vi "Auto Check Each Tube Posibly Modded for Prevent Trip.vi"(6 "error in (no error)":errorcluster, 8 "BoardHandle in":T1, 9 "Barcodes in":string[](array[string]), 10 "Tube #":i32) -> (0 "BoardHandle out":T1, 1 "error out":errorcluster, 2 "channel 4 currents":dbl[](array[numeric]), 3 "Actual Voltage Level (V) 2":dbl format="%#_13g", 5 "channel 3 currents":dbl[](array[numeric]), 7 "channel 2 currents":dbl[](array[numeric]), 11 "channel 1 currents":dbl[](array[numeric]))   [LabVIEW 2020]
uses:
  <instrlib>/CAEN PSM/CAEN PSM.lvlib
panel:
  # "OUTPUTS"
  # "INPUTS"
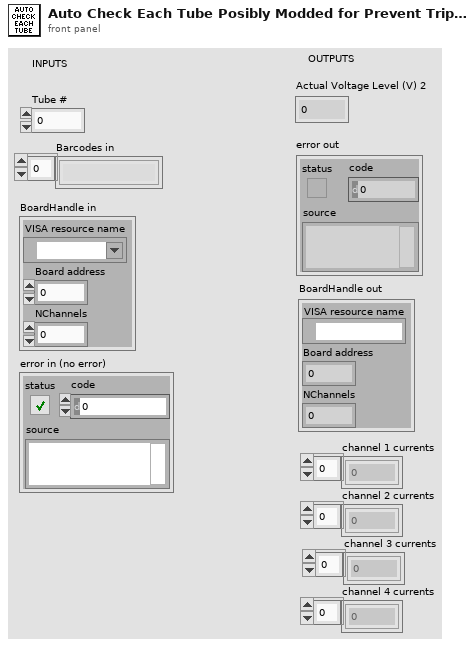
[diagram p1: front panel]
types:
  T1 = cluster{"VISA resource name":refnum<visa-resource-name>, "Board address":u8, "NChannels":u8}
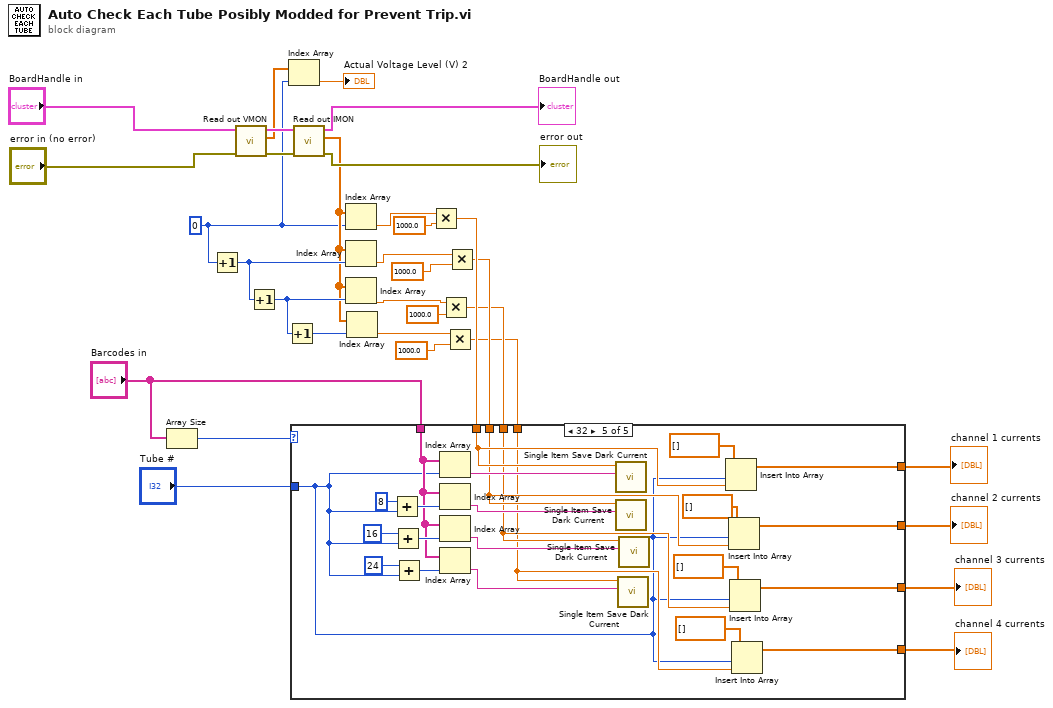
[diagram p0: block diagram]
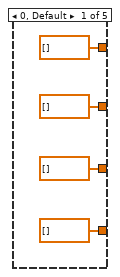
[diagram p2: hidden frame]
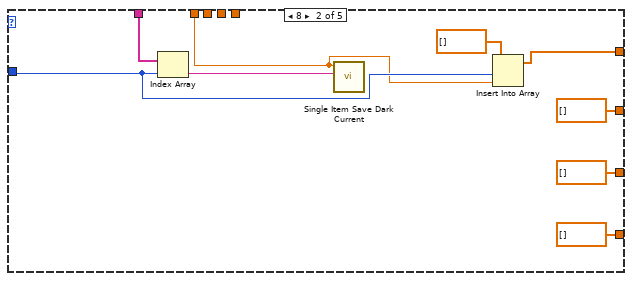
[diagram p3: hidden frame]
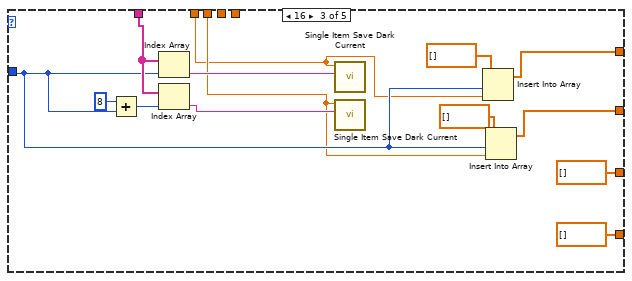
[diagram p4: hidden frame]
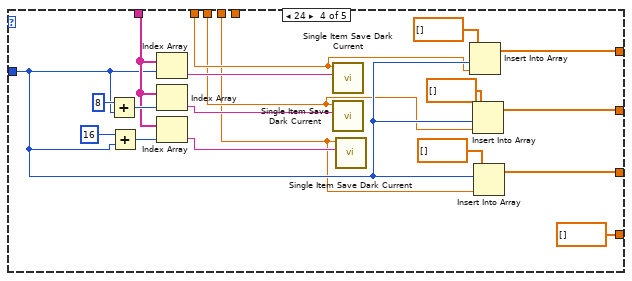
[diagram p5: hidden frame]
diagram:
  w18 = 0 ("index")
  n1 = Array Size(array="Barcodes in") -> (size(s)=w17:i32)
  n2 = Increment(x=w18) -> (x+1=w21:i32)
  n3 = call <instrlib>:"Read out VMON.vi"("error in (no error)"="error in (no error)", "BoardHandle"="BoardHandle in") -> ("error out"=w29:errorcluster, "VMon values (V)"=w27:dbl[], "BoardHandle out"=w28:T1)  [unwired: 7 in]
  n4 = Increment(x=w21) -> (x+1=w20:i32)
  n5 = Increment(x=w20) -> (x+1=w22:i32)
  n6 = Index Array(array=w27, index=w18) -> (element=→"Actual Voltage Level (V) 2":dbl)
  n7 = call <instrlib>:"Read out IMON.vi"("error in (no error)"=w29, "BoardHandle"=w28) -> ("error out"=→"error out":errorcluster, "IMon values (uA)"=w19:dbl[], "BoardHandle out"=→"BoardHandle out":T1)  [unwired: 6 in, 1 out]
  n8 = Index Array(array=w19, index=w18) -> (element=w30:dbl)
  n9 = Index Array(array=w19, index=w21) -> (element=w13:dbl)
  n10 = Index Array(array=w19, index=w20) -> (element=w9:dbl)
  n11 = Index Array(array=w19, index=w22) -> (element=w7:dbl)
  n12 = Multiply(x=w30, y=1000.0) -> (x*y=w16:dbl)
  n13 = Multiply(x=w9, y=1000.0) -> (x*y=w8:dbl)
  n14 = Multiply(x=w7, y=1000.0) -> (x*y=w5:dbl)
  n15 = Multiply(x=w13, y=1000.0) -> (x*y=w11:dbl)
  n16 = case shown="32" w17 {
    tunnel: w5 -> [_ _ _ _ w84]
    tunnel: w8 -> [_ _ _ w64 w86]
    tunnel: w11 -> [_ _ w51 w65 w88]
    tunnel: w16 -> [_ w41 w50 w66 w90]
    tunnel: "Barcodes in" -> [_ w44 w56 w73 w95]
    tunnel: "Tube #" -> [_ w42 w52 w67 w83]
    tunnel: [dbl[] [] ("array") w40 w49 w63 w82] -> w4
    tunnel: [dbl[] [] ("array") dbl[] [] ("array") w48 w62 w81] -> w3
    tunnel: [dbl[] [] ("array") dbl[] [] ("array") dbl[] [] ("array") w61 w80] -> w2
    tunnel: [dbl[] [] ("array") dbl[] [] ("array") dbl[] [] ("array") dbl[] [] ("array") w79] -> w1
    frame 0, Default {
    }
    frame 8 {
      n17 = Index Array(array=w44, index=w42) -> (element=w45:string)
      n18 = call "Single Item Save Dark Current.vi"("String"=w45, "Numeric"=w41) -> ()  [unwired: 10 in]
      n19 = Insert Into Array(array=dbl[] [], index=w42, new element=w41) -> (w40:dbl[])
    }
    frame 16 {
      n20 = Add(x=8, y=w52) -> (x+y=w59:i32)
      n21 = Index Array(array=w56, index=w52) -> (element=w57:string)
      n22 = Index Array(array=w56, index=w59) -> (element=w55:string)
      n23 = call "Single Item Save Dark Current.vi"("String"=w57, "Numeric"=w50) -> ()  [unwired: 10 in]
      n24 = call "Single Item Save Dark Current.vi"("String"=w55, "Numeric"=w51) -> ()  [unwired: 10 in]
      n25 = Insert Into Array(array=dbl[] [], index=w52, new element=w50) -> (w49:dbl[])
      n26 = Insert Into Array(array=dbl[] [], index=w52, new element=w51) -> (w48:dbl[])
    }
    frame 24 {
      n27 = Add(x=8, y=w67) -> (x+y=w78:i32)
      n28 = Add(x=16, y=w67) -> (x+y=w76:i32)
      n29 = Index Array(array=w73, index=w67) -> (element=w74:string)
      n30 = Index Array(array=w73, index=w78) -> (element=w72:string)
      n31 = Index Array(array=w73, index=w76) -> (element=w71:string)
      n32 = call "Single Item Save Dark Current.vi"("String"=w74, "Numeric"=w66) -> ()  [unwired: 10 in]
      n33 = call "Single Item Save Dark Current.vi"("String"=w72, "Numeric"=w65) -> ()  [unwired: 10 in]
      n34 = call "Single Item Save Dark Current.vi"("String"=w71, "Numeric"=w64) -> ()  [unwired: 10 in]
      n35 = Insert Into Array(array=dbl[] [], index=w67, new element=w66) -> (w63:dbl[])
      n36 = Insert Into Array(array=dbl[] [], index=w67, new element=w65) -> (w62:dbl[])
      n37 = Insert Into Array(array=dbl[] [], index=w67, new element=w64) -> (w61:dbl[])
    }
    frame 32 {
      n38 = Add(x=8, y=w83) -> (x+y=w102:i32)
      n39 = Add(x=16, y=w83) -> (x+y=w100:i32)
      n40 = Add(x=24, y=w83) -> (x+y=w98:i32)
      n41 = Index Array(array=w95, index=w83) -> (element=w96:string)
      n42 = Index Array(array=w95, index=w102) -> (element=w94:string)
      n43 = Index Array(array=w95, index=w100) -> (element=w93:string)
      n44 = Index Array(array=w95, index=w98) -> (element=w92:string)
      n45 = call "Single Item Save Dark Current.vi"("String"=w96, "Numeric"=w90) -> ()  [unwired: 10 in]
      n46 = call "Single Item Save Dark Current.vi"("String"=w94, "Numeric"=w88) -> ()  [unwired: 10 in]
      n47 = call "Single Item Save Dark Current.vi"("String"=w92, "Numeric"=w84) -> ()  [unwired: 10 in]
      n48 = call "Single Item Save Dark Current.vi"("String"=w93, "Numeric"=w86) -> ()  [unwired: 10 in]
      n49 = Insert Into Array(array=dbl[] [], index=w83, new element=w90) -> (w82:dbl[])
      n50 = Insert Into Array(array=dbl[] [], index=w83, new element=w88) -> (w81:dbl[])
      n51 = Insert Into Array(array=dbl[] [], index=w83, new element=w86) -> (w80:dbl[])
      n52 = Insert Into Array(array=dbl[] [], index=w83, new element=w84) -> (w79:dbl[])
    }
  }
  "channel 1 currents" <- w4
  "channel 2 currents" <- w3
  "channel 3 currents" <- w2
  "channel 4 currents" <- w1
